vi "String to U32.vi"(8 "error in":errorcluster, 11 "Integer String":string) -> (0 "error out":errorcluster, 3 "U32":u32)   [LabVIEW 2024, in "Electronic Datasheet.lvlib"]
doc: "Converts the string representation of a number in a specified base to an equivalent 32-bit unsigned integer."
uses:
  Core/Electronic Datasheet.lvlib
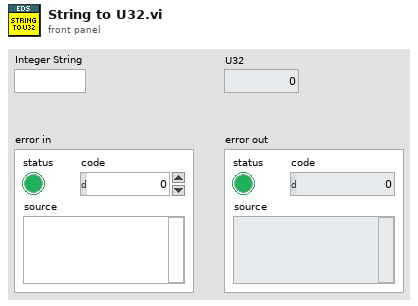
[diagram p1: front panel]
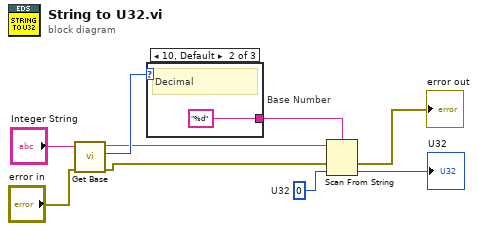
[diagram p0: block diagram]
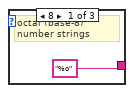
[diagram p2: hidden frame]
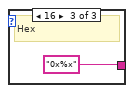
[diagram p3: hidden frame]
diagram:
  w8 = u32 0  # U32
  n1 = call "Get Base.vi"("error in"="error in", "Default Value"="Integer String") -> ("error out"=w2:errorcluster, "Number Base"=w9:u8, "Default Value (dup)"=w6:string)  [unwired: 7 in]
  n2 = case "Base Number" shown="10, Default" w9 {
    tunnel: ["%o" ("format string") "%d" ("format string") "0x%x" ("format string")] -> w7
    frame 8 {
      # "octal (base-8) number strings"
    }
    frame 10, Default {
      # "Decimal"
    }
    frame 16 {
      # "Hex"
    }
  }
  n3 = Scan From String(format string=w7, input string=w6, error in=w2, default 1=w8) -> (error out=→"error out":errorcluster, output 1=→"U32":u32)  [unwired: 1 in, 2 out]
